vi "Motor_Sim.vi"() -> ()   [LabVIEW 2014]
uses:
  <vilib>/Simulation/Scripting/Companion Diagram/SimConfigNode/SimParams.ctl
  <vilib>/Simulation/Scripting/Companion Diagram/SimConfigNode/_simSolvers.ctl
  <vilib>/Simulation/Implementation/Shared/SIMSCR Execution Mode.ctl
  <vilib>/Simulation/Param Hierarchy/Typedefs/SIMPH Param Control Actions.ctl
  <vilib>/Simulation/Implementation/Shared/NILVSim_ParamChanged.vi
  <vilib>/Simulation/Implementation/Shared/NILVSIM_BeginStep.vi
  <vilib>/Simulation/DataSources/Implementation/NILVSim Step.llb/SIM Step (scalar).vi
  <vilib>/Simulation/SignalDisplay/Implementation/NILVSim Time Waveform.llb/SIM Time Waveform (scalar).vi
  <vilib>/Simulation/Implementation/Shared/NILVSim_Manager.vi
  <vilib>/Utility/error.llb/Clear Errors.vi
  <vilib>/Simulation/Implementation/Shared/NILVSim_FinalizeModel.vi
  <vilib>/Simulation/Implementation/Shared/SIM Unbundle Sim Info.vi
  <vilib>/Simulation/Implementation/Shared/NILVSim_Initialize.vi
  <vilib>/Simulation/Utility/Implementation/NILVSim Get Time and IsAcceptedStep.vi
  <vilib>/Simulation/Implementation/Shared/SIMSH Read Queue.vi
  <vilib>/Simulation/Implementation/Shared/NILVSim_GetModelError.vi
  <vilib>/Simulation/Implementation/Shared/SIM Bundle Sim Info.vi
  <vilib>/Simulation/Scripting/Companion Diagram/SimConfigNode/SimDog.xnode
  Motor_subsys.vi
  <vilib>/Simulation/Implementation/XNodeFramework/SimXNode/SimX.xnode
  <vilib>/Simulation/Implementation/Shared/NI_SIM_Implementation.lvlib
panel:
  in  "Duty Cycle":dbl=1.0
  out "d_theta":dbl=400.4492509480051
  out "Angular Velocity":waveform(dbl)(graph)={"t0"=timestamp(0.5 s since 1904-01-01), "dt"=1.0, "Y"=[400.4492509480051]}
  out "Angle":waveform(dbl)(graph)={"t0"=timestamp(0.5 s since 1904-01-01), "dt"=1.0, "Y"=[186.16192312088987]}
  in  "R [ohm]":dbl=4.0
  in  "B [Nms]":dbl=1.65e-05
  in  "K [Nm/Amp]":dbl=0.0208
  in  "J [kg*m^2]":dbl=3.129e-06
  in  "L [H]":dbl=0.000514
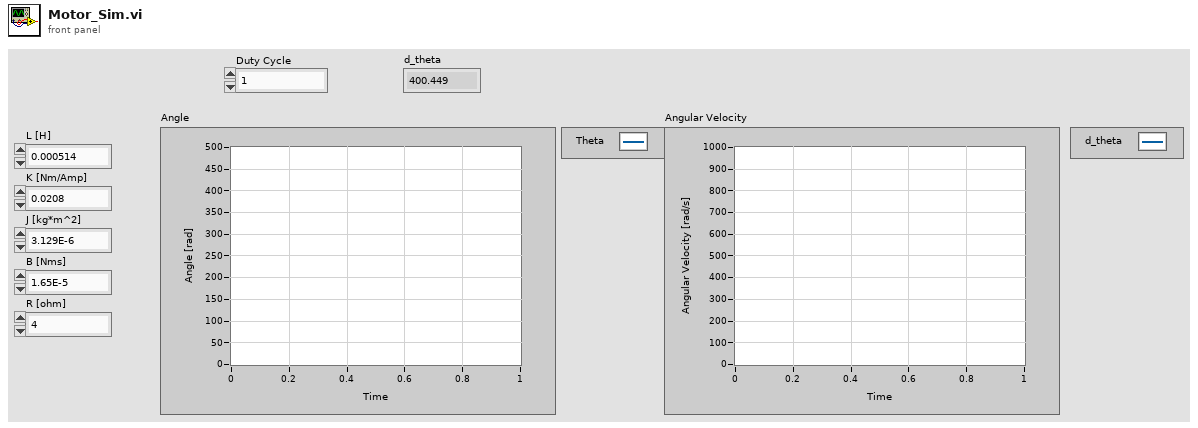
[diagram p1: front panel]
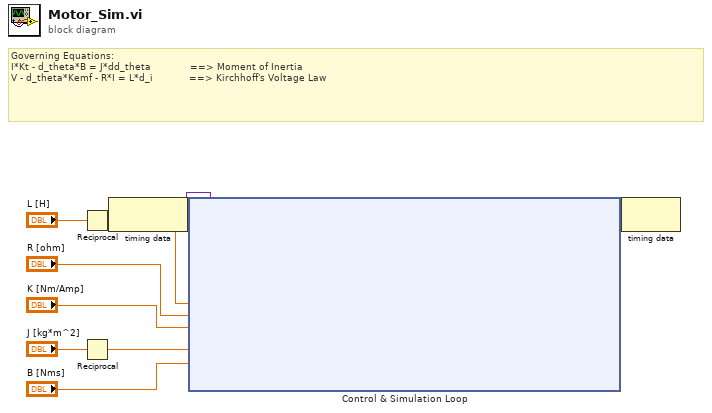
[diagram p0: block diagram]
diagram:
  # "Governing Equations: \nI*Kt - d_theta*B = J*dd_theta             ==> Moment of Inertia\nV - d_theta*Kemf - R*I = L*d_i            ==> Kirchhoff's Voltage Law"
  n1 = Reciprocal(x="L [H]") -> (1/x=w6:dbl)
  n2 = Reciprocal(x="J [kg*m^2]") -> (1/x=w4:dbl)
  n3 = node-c288() -> (w9:variant)  [unwired: 1 in]
  n4 = node-c254 "Control & Simulation Loop"(w9, w6, w4, "K [Nm/Amp]", "B [Nms]", "R [ohm]") -> (w8:variant)
  n5 = node-c288(w8) -> ()  [unwired: 1 out]
